vi "to Seconds.vi"(1 "Minute":i32, 2 "Second":i32, 3 "Hour":i32) -> (0 "Total Seconds":i32)   [LabVIEW 2020]
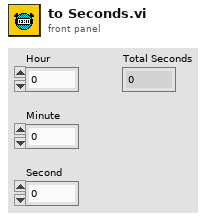
[diagram p1: front panel]
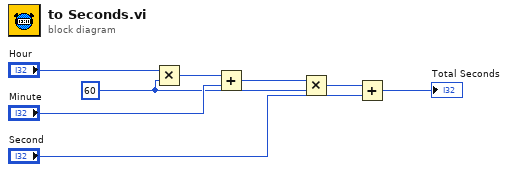
[diagram p0: block diagram]
diagram:
  w3 = 60 ("y")
  n1 = Multiply(x="Hour", y=w3) -> (x*y=w2:i32)
  n2 = Add(x=w2, y="Minute") -> (x+y=w4:i32)
  n3 = Multiply(x=w4, y=w3) -> (x*y=w6:i32)
  n4 = Add(x=w6, y="Second") -> (x+y=→"Total Seconds":i32)
